vi "Status Ramp.vi"(0 "VISA resource name":refnum<visa-resource-name>, 5 "Loop (0: 1)":u16(ring) items=["1", "2"], 11 "error in (no error)":errorcluster) -> (4 "VISA resource name out":refnum<visa-resource-name>, 6 "Ramping On/Off":bool, 8 "Rate Value":dbl min=0.0 max=100.0 step=0.001 format="%.3f", 10 "Ramping Active/Inactive":bool, 15 "error out":errorcluster)   [LabVIEW 2013, in "Lake Shore Cryotronics 331.lvlib"]
doc: "This VI displays the parameters of a control loop's ramp."
uses:
  Lake Shore Cryotronics 331.lvlib
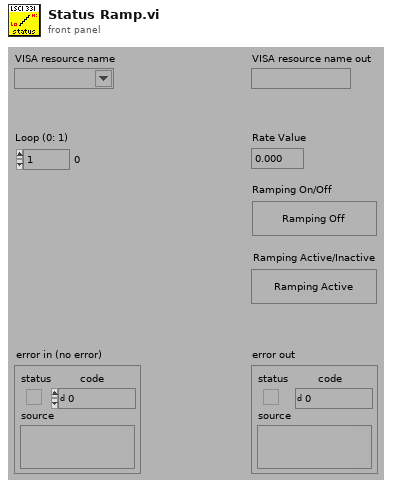
[diagram p1: front panel]
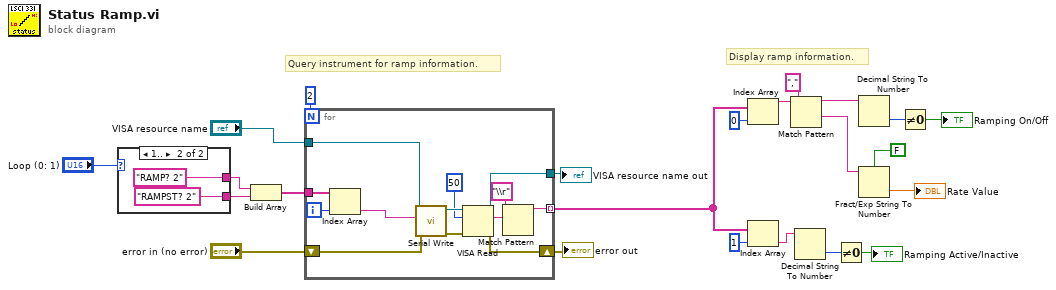
[diagram p0: block diagram]
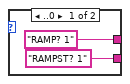
[diagram p2: hidden frame]
diagram:
  # "Display ramp information."
  # "Query instrument for ramp information."
  n1 = case shown="1.." "Loop (0: 1)" {
    tunnel: ["RAMPST? 1" "RAMPST? 2"] -> w17
    tunnel: ["RAMP? 1" "RAMP? 2"] -> w16
    frame ..0 {
    }
    frame 1.. {
    }
  }
  n2 = Build Array(w16, w17) -> (w18:string[])
  n3 = for {
    N: 2 -> [_]
    tunnel: w18 -> [w36]
    shift-right: [w33] -> w22
    shift-left: "error in (no error)" -> [w34]
    tunnel: [w32] -> w23
    tunnel: [w30] -> w2 mode=indexing
    tunnel: "VISA resource name" -> [w29]
    i -> [w35]
    n4 = Index Array(array=w36, index=w35) -> (element=w28:string)
    n5 = call "Serial Write.vi"("error in (no error)"=w34, "Write Buffer (\"\")"=w28, "VISA resource name"=w29) -> ("error out"=w39:errorcluster, "VISA resource name out"=w40:refnum<visa-resource-name>)  [unwired: 6 in, 1 out]
    n6 = VISA Read(VISA resource name=w40, byte count=50, error in (no error)=w39) -> (VISA resource name out=w32:refnum<visa-resource-name>, read buffer=w37:string, error out=w33:errorcluster)  [unwired: 1 out]
    n7 = Match Pattern(string=w37, regular expression="\\r") -> (before substring=w30:string)  [unwired: 1 in, 3 out]
  }
  "VISA resource name out" <- w23
  "error out" <- w22
  n8 = Index Array(array=w2, index=0) -> (element=w12:string)
  n9 = Index Array(array=w2, index=1) -> (element=w4:string)
  n10 = Match Pattern(string=w12, regular expression=",") -> (before substring=w11:string, after substring=w8:string)  [unwired: 1 in, 2 out]
  n11 = Decimal String To Number(string=w4) -> (number=w5:i32)  [unwired: 2 in, 1 out]
  n12 = Not Equal To 0?(x=w5) -> (x != 0?=→"Ramping Active/Inactive":bool)
  n13 = Decimal String To Number(string=w11) -> (number=w10:i32)  [unwired: 2 in, 1 out]
  n14 = Fract/Exp String To Number(use system decimal point (T)=FALSE, string=w8) -> (number=→"Rate Value":dbl)  [unwired: 2 in, 1 out]
  n15 = Not Equal To 0?(x=w10) -> (x != 0?=→"Ramping On/Off":bool)
